vi "ReadHexapodFile.vi"(4 "error in (not an error)":errorcluster, 7 "file path (use dialog)":path) -> (0 "error out":errorcluster, 3 "WaveformsHexapode":waveform(dbl)[](graph))   [LabVIEW 2017]
uses:
  <vilib>/regexp/Match Regular Expression.xnode
panel:
  out "subarray":string[](array[string])
  out "taille(s)":i32[](array[numeric])
  out "sous-tableau":dbl[][](array[numeric])
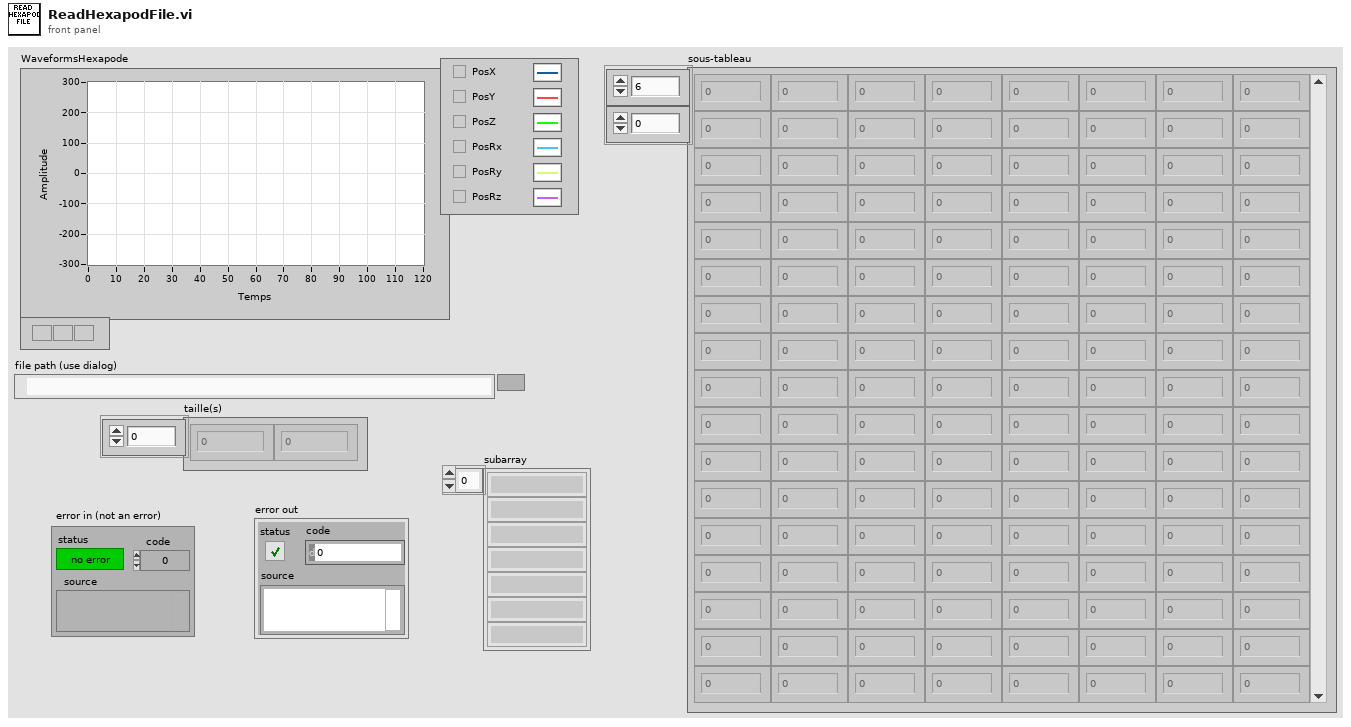
[diagram p1: front panel]
types:
  T1 = enum16{"open", "replace", "create", "open or create", "replace or create", "replace or create with confirmation"}
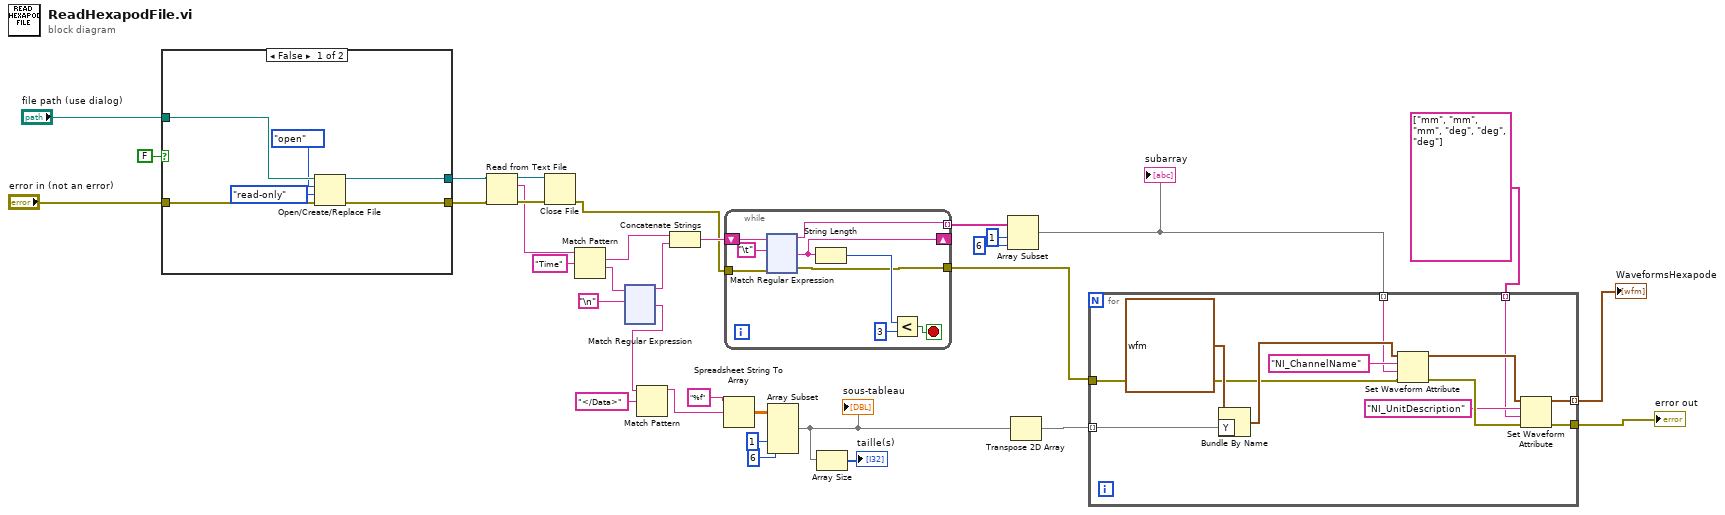
[diagram p0: block diagram]
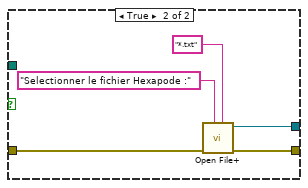
[diagram p2: hidden frame]
diagram:
  n1 = case shown="False" FALSE {
    tunnel: [w37 w42] -> w6
    tunnel: [w38 w41] -> w5
    tunnel: "error in (not an error)" -> [w39 w40]
    tunnel: "file path (use dialog)" -> [w36 _]
    frame False {
      n2 = Open/Create/Replace File(file path (use dialog)=w36, error in=w39, operation (0:open)=T1."open", access (0:read/write)=enum16{"read/write", "read-only", "write-only"}."read-only") -> (refnum out=w37:refnum<file>, error out=w38:errorcluster)  [unwired: 2 in, 1 out]
    }
    frame True {
      n3 = call <vilib>:"Open File+.vi"("[pattern]"="*.txt", "prompt"="Selectionner le fichier Hexapode :", "error in (not an error)"=w40) -> ("error out"=w41:errorcluster, "refnum"=w42:refnum<file>)  [unwired: 5 in, 2 out]
    }
  }
  n4 = Read from Text File(file (use dialog)=w6, error in=w5) -> (refnum out=w32:refnum<file>, text=w30:string, error out=w33:errorcluster)  [unwired: 2 in, 1 out]
  n5 = Close File(refnum=w32, error in=w33) -> (error out=w17:errorcluster)  [unwired: 1 out]
  n6 = Match Pattern(string=w30, regular expression="Time" ("expression régulière")) -> (match substring=w22:string, after substring=w28:string)  [unwired: 1 in, 2 out]
  n7 = xnode "Match Regular Expression"("chaîne en entrée"=w28, "expression régulière"="\n") -> ("avant la correspondance"=w23:string, "après la correspondance"=w9:string)  [unwired: 4 in, 3 out]
  n8 = Match Pattern(string=w9, regular expression="</Data>" ("expression régulière")) -> (before substring=w7:string)  [unwired: 1 in, 3 out]
  n9 = Concatenate Strings(w22, w23) -> (w21:string)
  n10 = Spreadsheet String To Array(format string="%f" ("séparateur (Tabulation)"), spreadsheet string=w7) -> (array=w26:dbl[][])  [unwired: 2 in]
  n11 = while {
    shift-right: [w48] -> _
    shift-left: w21 -> [w52]
    tunnel: [w47] -> w13 mode=indexing
    tunnel: w17 -> [w46]
    tunnel: [w45] -> w16
    stop <- w51 stop-if-true
    n12 = xnode "Match Regular Expression"("chaîne en entrée"=w52, "expression régulière"="\t", "entrée d'erreur"=w46) -> ("avant la correspondance"=w47:string, "après la correspondance"=w48:string, "sortie d'erreur"=w45:errorcluster)  [unwired: 3 in, 2 out]
    n13 = String Length(string=w48) -> (length=w50:i32)
    n14 = Less?(x=w50, y=3) -> (x < y?=w51:bool)
  }
  n15 = Array Subset(array=w26, index (col)=1 ("indice"), length (col)=6 ("longueur")) -> (w11:dbl[][])  [unwired: 2 in]
  "sous-tableau" <- w11
  n16 = Array Size(array=w11) -> (size(s)=→"taille(s)":i32[])
  n17 = Array Subset(array=w13, index=1 ("indice"), length=6 ("longueur")) -> (w12:string[])
  "subarray" <- w12
  n18 = Transpose 2D Array(2D array=w11) -> (transposed array=w18:dbl[][])
  n19 = for {
    tunnel: w18 -> [w175] mode=indexing
    tunnel: w16 -> [w169]
    tunnel: w12 -> [w168] mode=indexing
    tunnel: string[] ["mm", "mm", "mm", "deg", "deg", "deg"] -> [w167] mode=indexing
    tunnel: [w166] -> w14 mode=indexing
    tunnel: [w165] -> w3
    n20 = Bundle By Name(cluster=waveform(dbl) {"t0"=timestamp(0 s since 1904-01-01), "dt"=0.01, "Y"=[]} ("waveform"), "Y"=w175) -> (w170:waveform(dbl))
    n21 = Set Waveform Attribute(4:w169, 5:w168, 6:"NI_ChannelName" ("nom"), 7:w170) -> (0:w173:errorcluster, 3:w174:waveform(dbl))  [unwired: 1 out]
    n22 = Set Waveform Attribute(4:w173, 5:w167, 6:"NI_UnitDescription" ("nom"), 7:w174) -> (0:w165:errorcluster, 3:w166:waveform(dbl))  [unwired: 1 out]
  }
  "WaveformsHexapode" <- w14
  "error out" <- w3
